vi "Get Hi Low Times Out Hum V.vi"(8 "error in (no error)":errorcluster, 10 "DateTimeLowOutHum":T1, 11 "DateTimeHiOutHum":T1) -> (0 "error out":errorcluster, 1 "function return":i16, 2 "DateTimeLowOutHum out":T1, 3 "DateTimeHiOutHum out":T1)   [LabVIEW 2009, in "VantagePro.lvlib"]
doc: "DllAccess short int _stdcall GetHiLowTimesOutHum_V (DateTime* DateTimeHiOutHum, DateTime* DateTimeLowOutHum);"
uses:
  VantagePro.lvlib
  <userlib>/VantagePro/VantagePro.dll
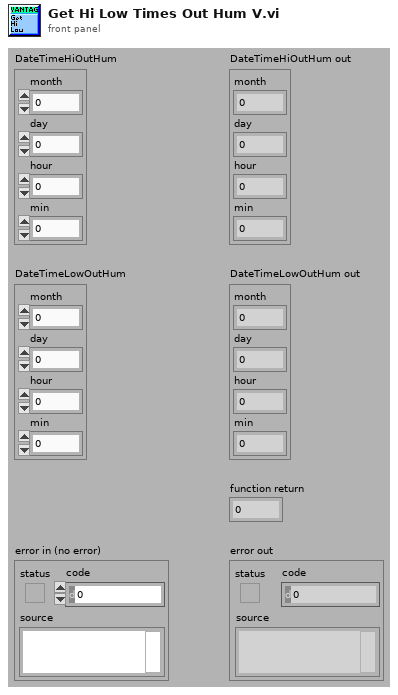
[diagram p1: front panel]
types:
  T1 = cluster{"month":i16, "day":i16, "hour":i16, "min":i16}
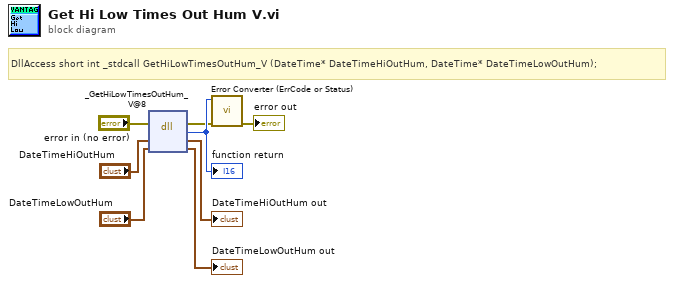
[diagram p0: block diagram]
diagram:
  # "DllAccess short int _stdcall GetHiLowTimesOutHum_V (DateTime* DateTimeHiOutHum, DateTime* DateTimeLowOutHum);"
  n1 = dll-call lib="C:/Program Files/National Instruments/LabVIEW 2010/user.lib/VantagePro/VantagePro.*" fn="_GetHiLowTimesOutHum_V@8"(error in="error in (no error)", "DateTimeHiOutHum"="DateTimeHiOutHum", "DateTimeLowOutHum"="DateTimeLowOutHum") -> (error out=w2:errorcluster, w8:i16, "DateTimeHiOutHum"=→"DateTimeHiOutHum out":T1, "DateTimeLowOutHum"=→"DateTimeLowOutHum out":T1)  [unwired: 2 in, 1 out]
  "function return" <- w8
  n2 = call "Error Converter (ErrCode or Status).vi"("error in (no error)"=w2, "error code"=w8) -> ("error out"=→"error out":errorcluster)  [unwired: 9 in]
